vi "Counter reset.vi"(5 "RESET":bool, 7 "IP":string="192.168.23.100", 8 "error in (no error)":errorcluster, 10 "PORT":i32 min=0 max=4 step=1, 11 "MASTER":i32 min=0 max=10 step=1) -> (0 "error out":errorcluster)   [LabVIEW 2022 SP3]
uses:
  <vilib>/NI/Advanced HTTP Client/POST (Buffer).vi
  <vilib>/NI/Advanced HTTP Client/Session.lvclass
panel:
  # "Reset user counter"
  # "Only resettable counter (2) index 82"
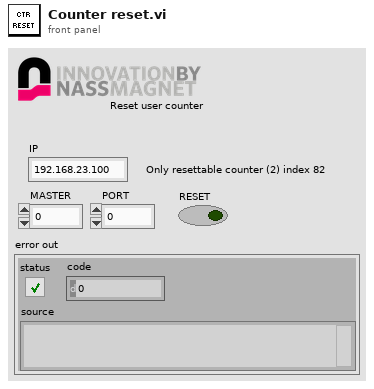
[diagram p1: front panel]
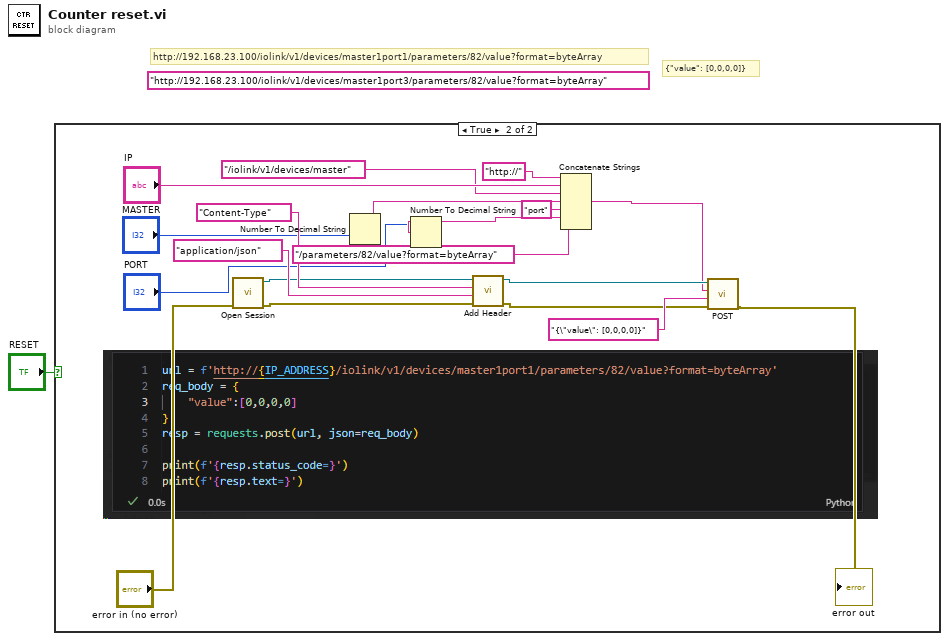
[diagram p0: block diagram]
diagram:
  (unwired) "http://192.168.23.100/iolink/v1/devices/master1port3/parameters/82/value?format=byteArray" ("url")
  # "http://192.168.23.100/iolink/v1/devices/master1port1/parameters/82/value?format=byteArray"
  # "{\"value\": [0,0,0,0]}"
  n1 = case shown="True" "RESET" {
    frame False {
    }
    frame True {
      n2 = call <vilib>:"Open Session.vi"("error in"="error in (no error)") -> ("error out"=w14:errorcluster, "session"=w15:refnum<class "Session.lvclass">)  [unwired: 9 in]
      n3 = Number To Decimal String(number="MASTER") -> (decimal integer string=w8:string)  [unwired: 1 in]
      n4 = Number To Decimal String(number="PORT") -> (decimal integer string=w5:string)  [unwired: 1 in]
      n5 = call <vilib>:"Add Header.vi"("error in"=w14, "value"="application/json" ("buffer"), "header"="Content-Type", "session in"=w15) -> ("error out"=w16:errorcluster, "session out"=w20:refnum<class "Session.lvclass">)  [unwired: 6 in]
      n6 = Concatenate Strings("http://", "IP", "/iolink/v1/devices/master" ("string"), w8, "port" ("string"), w5, "/parameters/82/value?format=byteArray" ("string")) -> (w9:string)
      n7 = call-poly <vilib>:"POST.vi"("error in"=w16, "buffer"="{\"value\": [0,0,0,0]}", "url"=w9, "session in"=w20) -> ("error out"=→"error out":errorcluster)  [unwired: 3 in, 4 out]
    }
  }
